vi "CustomDeviceUI.vi"() -> ()   [LabVIEW 2015, in "CustomDevice.lvclass"]
uses:
  CustomDevice.lvclass
  <vilib>/NI/Configuration Framework/Node/NodeRef.ctl
  <vilib>/NI/Configuration Framework/Node/NISE_CEF_Node.lvclass
  <vilib>/NI/AMC/Message Queue.ctl
  <vilib>/NI/AMC/Message.ctl
  <vilib>/NI/Tools/Keyed Array/KeyedArray.ctl
  <vilib>/NI/Configuration Framework/Node/UserEventRef.ctl
  <vilib>/NI/Configuration Framework/Controls/EventCluster.ctl
  CustomDevice.lvclass/CustomDevice.ctl
  Read Main CD Properties.vi
  Write Main CD Properties.vi
  <vilib>/NI/AMC/Create Single Message.vi
  <vilib>/NI/AMC/Update Message Routing Info.vi
  <vilib>/NI/AMC/Send Message.vi
  <vilib>/NI/AMC/AMC.lvlib
  <vilib>/NI/Tools/Keyed Array/Tools_KeyedArray.lvlib
  <vilib>/NI/Configuration Framework/NISE_CEF_TreeControl.lvlib
panel:
  in  "Main Page GUID":string
  in  "Custom Device Type":T1(ring)
  in  "Version":string
  in  "Max Occurrences":i32
  in  "Custom Device Name":string
  in  "user event":T2
  in  "main queue":T3
  in  "node ref":T4
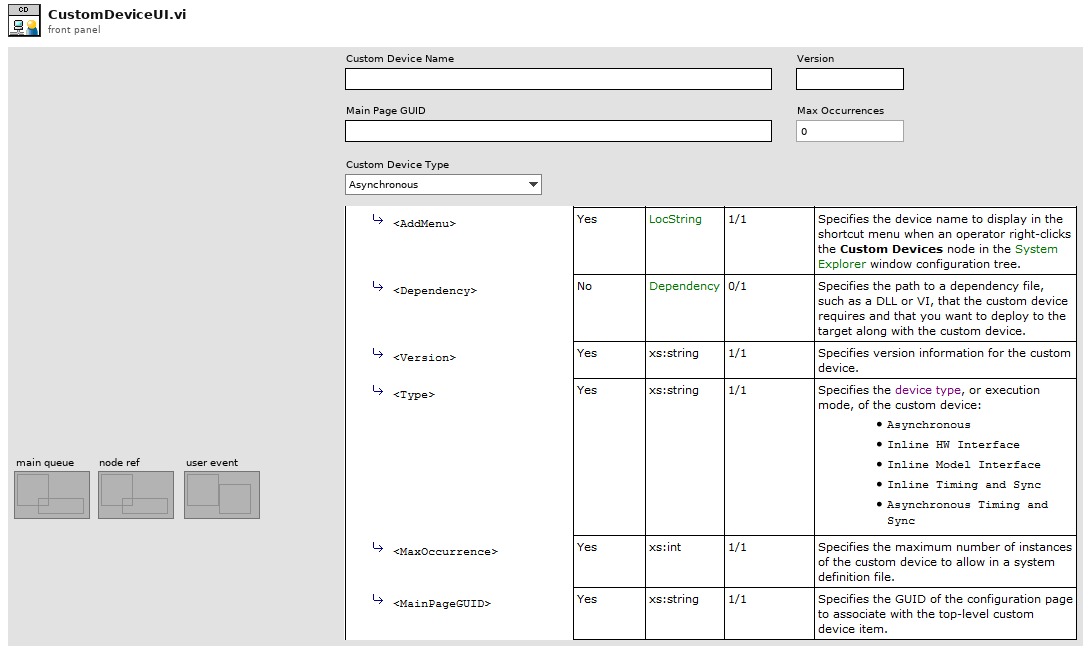
[diagram p1: front panel]
types:
  T1 = enum16{"Asynchronous", "Inline HW Interface", "Inline Model Interface", "Inline Timing and Sync", "Asynchronous Timing and Sync"}
  T2 = typedef "NISE_CEF_Node.lvclass/UserEventRef.ctl" = refnum<user-event>
  T3 = typedef "AMC.lvlib/Message Queue.ctl" = refnum<queue>
  T4 = typedef "NISE_CEF_Node.lvclass/NodeRef.ctl" = refnum<data-value>
  T5 = typedef "Main Custom Device Properties.ctl" = cluster{"CD Name":string, "Version":string, "Max Occurrences":i32, "Device Type":enum16{"Asynchronous", "Inline HW Interface", "Inline Model Interface", "Inline Timing and Sync", "Asynchronous Timing and Sync"}, "Main Page GUID":string}
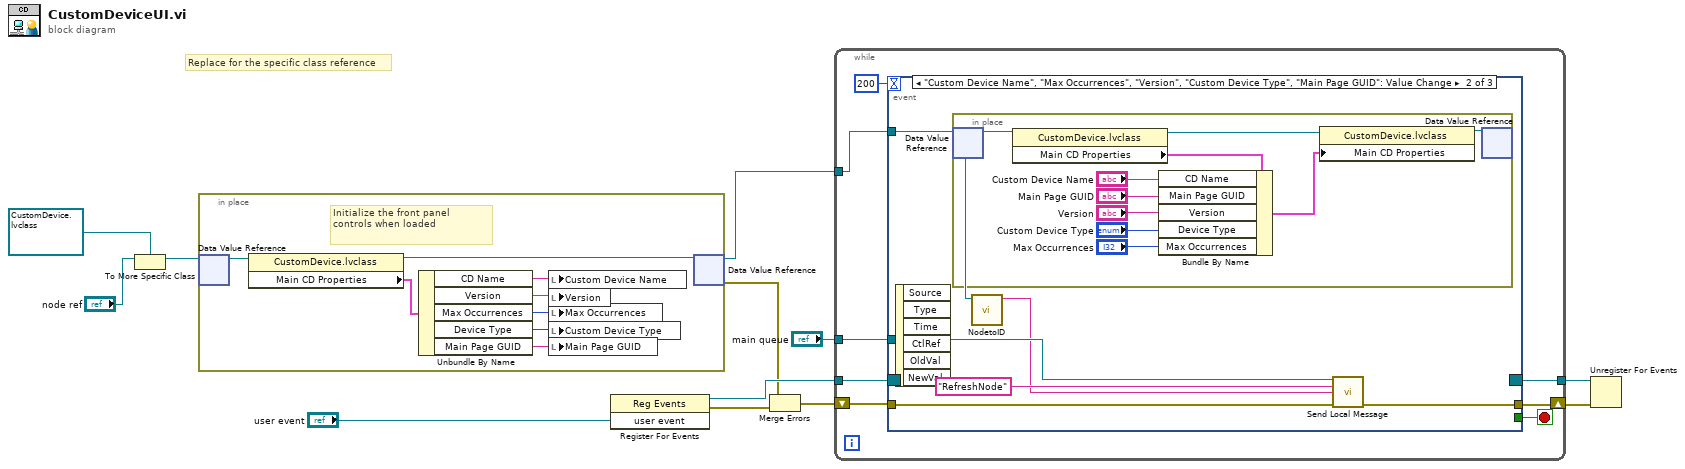
[diagram p0: block diagram]
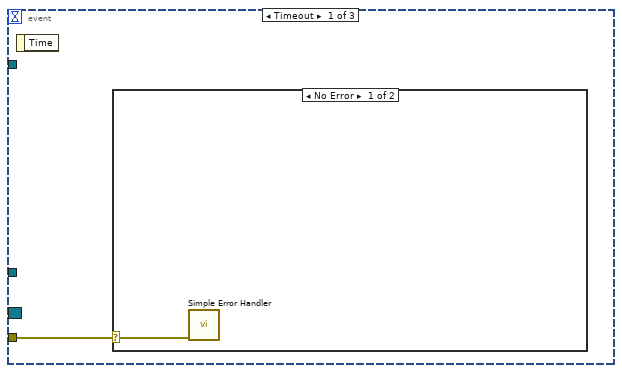
[diagram p2: hidden frame]
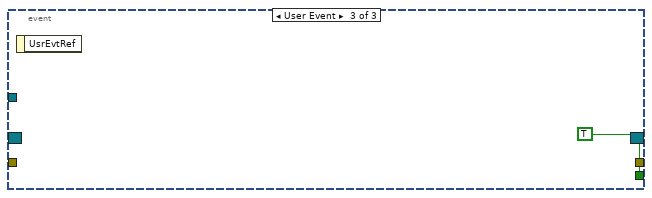
[diagram p4: hidden frame]
diagram:
  # "Replace for the specific class reference"
  n1 = To More Specific Class(target class=refnum<data-value> refnum ("data value reference"), reference="node ref") -> (specific class reference=w5:refnum<data-value>)  [unwired: 1 in, 1 out]
  n2 = in-place {
    # "Initialize the front panel controls when loaded"
    n3 = in-place-dvr #1(w5) -> (w20:refnum<class "CustomDevice.lvclass">)  [unwired: 1 out]
    n4 = property class="CustomDevice.lvclass"(reference=w20) -> (reference out=w19:refnum<class "CustomDevice.lvclass">, "Main CD Properties"=w18:T5)  [unwired: 1 in, 1 out]
    n5 = Unbundle By Name(w18) -> ("CD Name"=w17:string, "Version"=w16:string, "Max Occurrences"=w15:i32, "Device Type"=w14:T1, "Main Page GUID"=w13:string)
    n6 = local write "Custom Device Name"(w17) -> ()
    n7 = local write "Version"(w16) -> ()
    n8 = local write "Max Occurrences"(w15) -> ()
    n9 = local write "Custom Device Type"(w14) -> ()
    n10 = local write "Main Page GUID"(w13) -> ()
    n11 = in-place-dvr #1(w19) -> (w12:refnum<data-value>, w2:errorcluster)
  }
  n12 = register-events("user event") -> (reference out=w9:refnum<event-registration>, error out=w3:errorcluster)  [unwired: 2 in]
  n13 = Merge Errors(w2, w3) -> (w1:errorcluster)
  n14 = while {
    tunnel: w12 -> [w28]
    tunnel: "main queue" -> [w27]
    tunnel: w9 -> [w25]
    tunnel: [w24] -> w8
    shift-right: [w22] -> w7
    shift-left: w1 -> [w21]
    stop <- w23 stop-if-true
    n15 = event shown="[1] \"Custom Device Name\", \"Max Occurrences\", \"Version\", \"Custom Device Type\", \"Main Page GUID\": Value Change" {
      selector: w25 -> [_ _ _]
      dyn-events: [_ _ _] -> w24
      timeout: 200 -> [_ _ _]
      tunnel: w28 -> [_ w34 _]
      tunnel: w27 -> [_ w35 _]
      tunnel: [_ _ TRUE] -> w23
      tunnel: [_ w32 _] -> w22
      tunnel: w21 -> [w29 w31 _]
      event Timeout {
        n16 = event-data() -> ()  [unwired: 1 in, 1 out]
        n17 = case shown="No Error" w29 {
          selector: w29 -> [w30 _]
          frame No Error {
            n18 = call <vilib>:"Simple Error Handler.vi"("error in (no error)"=w30) -> ()  [unwired: 4 in, 5 out]
          }
          frame Error {
          }
        }
      }
      event "Custom Device Name", "Max Occurrences", "Version", "Custom Device Type", "Main Page GUID": Value Change {
        n19 = event-data() -> ()  [unwired: 1 in, 6 out]
        n20 = in-place {
          n21 = in-place-dvr #2(w34) -> (w45:refnum<class "CustomDevice.lvclass">)  [unwired: 1 out]
          n22 = property class="CustomDevice.lvclass"(reference=w45) -> (reference out=w44:refnum<class "CustomDevice.lvclass">, "Main CD Properties"=w43:T5)  [unwired: 1 in, 1 out]
          n23 = Bundle By Name(cluster=w43, "CD Name"="Custom Device Name", "Main Page GUID"="Main Page GUID", "Version"="Version", "Device Type"="Custom Device Type", "Max Occurrences"="Max Occurrences") -> (w42:T5)
          n24 = property class="CustomDevice.lvclass"(reference=w44, "Main CD Properties"=w42) -> (reference out=w46:refnum<class "CustomDevice.lvclass">)  [unwired: 1 in, 1 out]
          n25 = in-place-dvr #2(w46) -> ()  [unwired: 2 out]
        }
        n26 = call <vilib>:"NodetoID.vi"("node ref"=w34) -> ("ID"=w33:string)  [unwired: 9 in, 1 out]
        n27 = call <vilib>:"Send Local Message.vi"("message queue in"=w35, "message name"="RefreshNode" ("Message Name"), "message value"=w33, "error in"=w31) -> ("error out"=w32:errorcluster)  [unwired: 9 in, 2 out]
      }
      event User Event {
        n28 = event-data() -> ()  [unwired: 1 in, 1 out]
      }
    }
  }
  n29 = Unregister For Events(event registration refnum=w8, error in=w7) -> ()  [unwired: 1 out]
